vi "ultrasonic.vi"(11 "State":enum16{"Start", "Run", "Finish"}(ring)) -> (3 "Distance":dbl)   [LabVIEW 2014]
uses:
  <vilib>/Rock Robotics/SystemInterfaces/DIO/FPGA_DIOChannel.ctl
  <vilib>/Rock Robotics/WPI/Ultrasonic/WPI_SonarMB1010DigitalOpen.vi
  <vilib>/Rock Robotics/WPI/Ultrasonic/WPI_SonarMB1010DigitalGetRange.vi
  <vilib>/Rock Robotics/WPI/Ultrasonic/WPI_SonarMB1010DigitalClose.vi
panel:
  # "in inches"
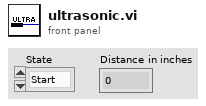
[diagram p1: front panel]
types:
  T1 = typedef "FPGA_DIOChannel.ctl" = enum8{"DIO 0", "DIO 1", "DIO 2", "DIO 3", "DIO 4", "DIO 5", "DIO 6", "DIO 7", "DIO 8", "DIO 9", "DIO MXP 0", "DIO MXP 1", "DIO MXP 2", "DIO MXP 3", "DIO MXP 4", "DIO MXP 5", "DIO MXP 6", "DIO MXP 7", "DIO MXP 8", "DIO MXP 9", "DIO MXP 10", "DIO MXP 11", "DIO MXP 12", "DIO MXP 13", "DIO MXP 14", "DIO MXP 15", "Invalid"}
  T2 = typedef "WPI_SonarMB1010DigitalDeviceRef.ctl" = cluster{"CounterDevRef":T3, "Scaling factor (s/in)":dbl}
  T3 = typedef "WPI_CounterDevRef.ctl" = cluster{"DevStatus":errorcluster, "CntIndex":T4}
  T4 = typedef "FPGA_CounterCtrSystemIndex.ctl" = enum8{"Ctr 0", "Ctr 1", "Ctr 2", "Ctr 3", "Ctr 4", "Ctr 5", "Ctr 6", "Ctr 7", "Invalid"}
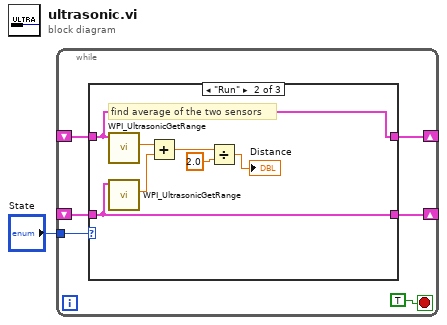
[diagram p0: block diagram]
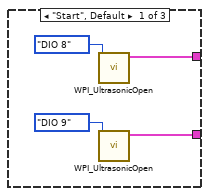
[diagram p2: hidden frame]
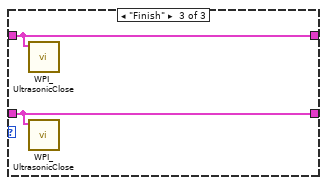
[diagram p3: hidden frame]
diagram:
  n1 = while {
    tunnel: "State" -> [w7]
    shift-right: [w5] -> _
    shift-left: _ -> [w3]
    shift-right: [w4] -> _
    shift-left: _ -> [w2]
    stop <- TRUE stop-if-true
    n2 = case shown="\"Run\"" w7 {
      tunnel: [w11 w16 w20] -> w5
      tunnel: [w10 w15 w19] -> w4
      tunnel: w3 -> [_ w16 w20]
      tunnel: w2 -> [_ w15 w19]
      frame "Start", Default {
        n3 = call-poly <vilib>:"WPI_UltrasonicOpen.vi"("DIO Channel"=FPGA_DIOChannel."DIO 8") -> ("SonarMB1010DigitalDevRef"=w11:T2)  [unwired: 9 in, 1 out]
        n4 = call-poly <vilib>:"WPI_UltrasonicOpen.vi"("DIO Channel"=FPGA_DIOChannel."DIO 9") -> ("SonarMB1010DigitalDevRef"=w10:T2)  [unwired: 9 in, 1 out]
      }
      frame "Run" {
        # "find average of the two sensors"
        n5 = call-poly <vilib>:"WPI_UltrasonicGetRange.vi"("SonarMB1010DigitalDevRef"=w16) -> ("Distance"=w14:dbl)  [unwired: 8 in, 2 out]
        n6 = call-poly <vilib>:"WPI_UltrasonicGetRange.vi"("SonarMB1010DigitalDevRef"=w15) -> ("Distance"=w13:dbl)  [unwired: 8 in, 2 out]
        n7 = Add(x=w14, y=w13) -> (x+y=w18:dbl)
        n8 = Divide(x=w18, y=2.0) -> (x/y=→"Distance":dbl)
      }
      frame "Finish" {
        n9 = call-poly <vilib>:"WPI_UltrasonicClose.vi"("SonarMB1010DigitalDevRef"=w20) -> ()  [unwired: 10 in, 1 out]
        n10 = call-poly <vilib>:"WPI_UltrasonicClose.vi"("SonarMB1010DigitalDevRef"=w19) -> ()  [unwired: 10 in, 1 out]
      }
    }
  }
